vi "test rotation.vi"() -> ()   [LabVIEW 2017]
panel:
  in  "Stop Button":bool
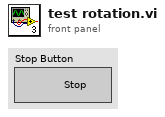
[diagram p1: front panel]
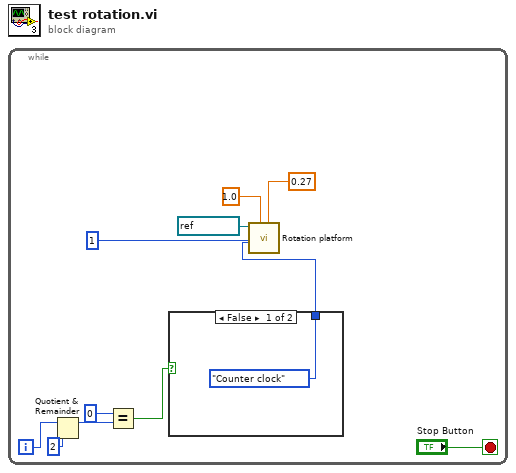
[diagram p0: block diagram]
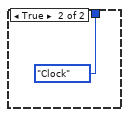
[diagram p2: hidden frame]
diagram:
  n1 = while {
    i -> [w6]
    stop <- "Stop Button" stop-if-true
    n2 = Quotient & Remainder(x=w6, y=2) -> (x-y*floor(x/y)=w4:i32)  [unwired: 1 out]
    n3 = Equal?(x=0, y=w4) -> (x = y?=w2:bool)
    n4 = case shown="False" w2 {
      tunnel: [enum16{"Counter clock", "Clock"}."Counter clock" ("Direction") enum16{"Counter clock", "Clock"}."Clock" ("Direction")] -> w1
      frame False {
      }
      frame True {
      }
    }
    n5 = call "Rotation platform.vi"("Revolution (0-0.5)"=0.27, "Rotation speed (RPM)"=1.0, "Direction"=w1, "Pump number"=1, "Rotation COM"=refnum<visa-resource-name> "COM7") -> ()  [unwired: 7 in]
  }
